vi "Setup Statically-Linked subWorkers.vi"(8 "error in":errorcluster, 11 "gRPC Client Tester in":refnum<class "gRPC Client Tester.lvclass">) -> (0 "error out":errorcluster, 3 "gRPC Client Tester out":refnum<class "gRPC Client Tester.lvclass">)   [LabVIEW 2019, in "gRPC Client Tester.lvclass"]
doc: "This VI performs a setup of all the statically-linked subWorkers that belong to the Worker that owns this VI. This VI must be called <b>before</b> any statically-linked subWorkers are called."
uses:
  gRPC Client Tester.lvclass
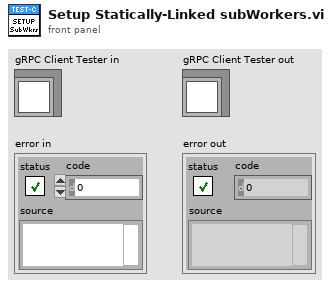
[diagram p1: front panel]
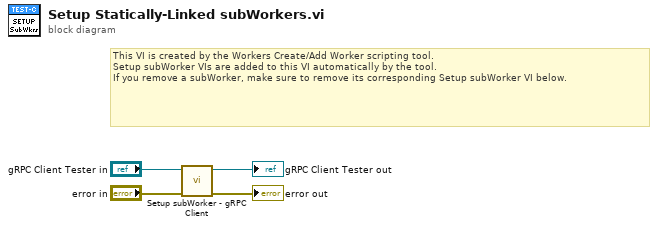
[diagram p0: block diagram]
diagram:
  # "This VI is created by the Workers Create/Add Worker scripting tool.\nSetup subWorker VIs are added to this VI automatically by the tool.\nIf you remove a subWorker, make sure to remove its corresponding Setup subWorker VI below."
  n1 = call "Setup subWorker - gRPC Client.vi"("error in"="error in", "gRPC Client Tester in"="gRPC Client Tester in") -> ("error out"=→"error out":errorcluster, "gRPC Client Tester out"=→"gRPC Client Tester out":refnum<class "gRPC Client Tester.lvclass">)  [unwired: 8 in]
